vi "Update Tree.vi"(10 "Parent Tag":string, 11 "Tree In":refnum<vi>) -> (3 "Tree Out":refnum<vi>)   [LabVIEW 2018, in "Tree Browser.lvlib"]
doc: "Update the child node of a tree. Tree contents won't be changed if the folders on disk match what's in the tree.\n\nNote that panel updates will be deferred while this VI runs, and the busy cursor set. Both are unset at completion of the VI."
uses:
  Tree Browser.lvlib
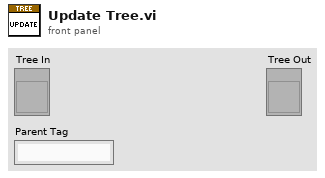
[diagram p1: front panel]
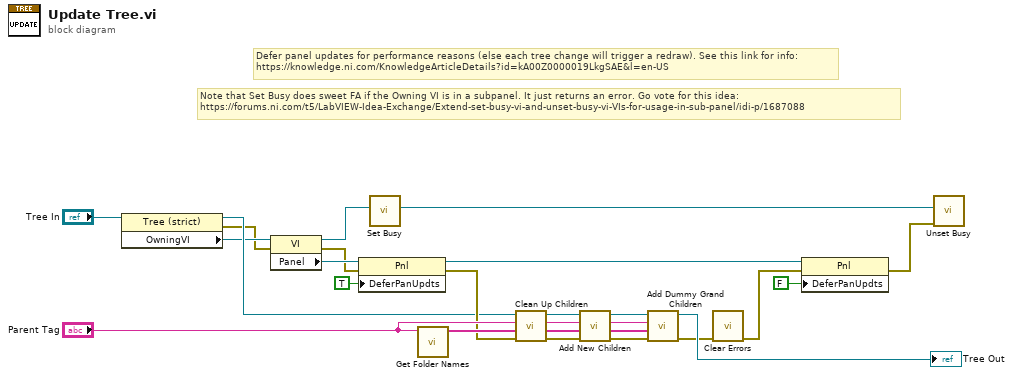
[diagram p0: block diagram]
diagram:
  # "Note that Set Busy does sweet FA if the Owning VI is in a subpanel. It just returns an error. Go vote for this idea:\nhttps://forums.ni.com/t5/LabVIEW-Idea-Exchange/Extend-set-busy-vi-and-unset-busy-vi-VIs-for-usage-in-sub-panel/idi-p/1687088"
  # "Defer panel updates for performance reasons (else each tree change will trigger a redraw). See this link for info:\nhttps://knowledge.ni.com/KnowledgeArticleDetails?id=kA00Z0000019LkgSAE&l=en-US"
  n1 = property class="Tree (strict)"(reference="Tree In") -> (reference out=w11:refnum<vi>, error out=w5:errorcluster, "OwningVI"=w7:refnum<vi>)  [unwired: 1 in]
  n2 = property class="VI"(reference=w7, error in=w5) -> (reference out=w3:refnum<vi>, error out=w4:errorcluster, "Panel"=w6:refnum<vi>)
  n3 = property class="Pnl"(reference=w6, error in=w4, "DeferPanUpdts"=TRUE ("Defer Panel Updates")) -> (reference out=w8:refnum<vi>, error out=w21:errorcluster)
  n4 = call <vilib>:"Set Busy.vi"("VI reference (current VI)"=w3) -> ()  [unwired: 9 in, 2 out]
  n5 = call "Get Folder Names.vi"("Parent Tag"="Parent Tag") -> ("Folder Names"=w22:string[])  [unwired: 10 in]
  n6 = call "Clean Up Children.vi"("error in (no error)"=w21, "Folder Names"=w22, "Parent Tag"="Parent Tag", "Tree In"=w11) -> ("error out"=w20:errorcluster, "Folder Names Dup"=w18:string[], "Parent Tag Dup"=w19:string, "Tree Out"=w17:refnum<vi>)  [unwired: 4 in]
  n7 = call "Add New Children.vi"("error in (no error)"=w20, "Folder Names"=w18, "Parent Tag"=w19, "Tree In"=w17) -> ("error out"=w14:errorcluster, "Folder Names Dup"=w13:string[], "Parent Tag Dup"=w15:string, "Tree Out"=w16:refnum<vi>)  [unwired: 4 in]
  n8 = call "Add Dummy Grand Children.vi"("error in (no error)"=w14, "Folder Names"=w13, "Parent Tag"=w15, "Tree In"=w16) -> ("error out"=w12:errorcluster, "Tree Out"=→"Tree Out":refnum<vi>)  [unwired: 4 in, 2 out]
  n9 = call <vilib>:"Clear Errors.vi"("error in (no error)"=w12) -> ("error out"=w1:errorcluster)  [unwired: 5 in, 1 out]
  n10 = property class="Pnl"(reference=w8, error in=w1, "DeferPanUpdts"=FALSE ("Defer Panel Updates")) -> (error out=w2:errorcluster)  [unwired: 1 out]
  n11 = call <vilib>:"Unset Busy.vi"("error in (no error)"=w2, "VI reference (current VI)"=w3) -> ()  [unwired: 9 in, 1 out]
